vi "WhileLoop.vi"() -> ()   [LabVIEW 2019]
panel:
  in  "milliseconds to wait":u32=500
  out "Waveform Chart":dbl(graph)=0.5543790091498753
  in  "stop":bool
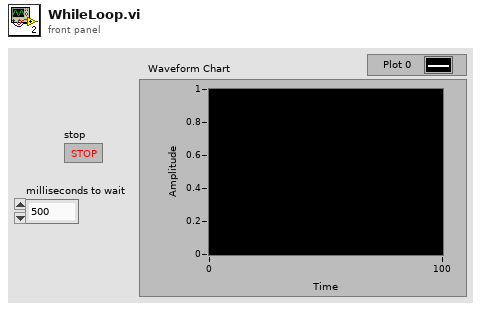
[diagram p1: front panel]
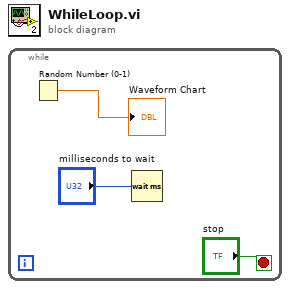
[diagram p0: block diagram]
diagram:
  n1 = while {
    stop <- "stop" stop-if-true
    n2 = Random Number (0-1)() -> (number: 0 to 1=→"Waveform Chart":dbl)
    n3 = Wait (ms)(milliseconds to wait="milliseconds to wait") -> ()  [unwired: 1 out]
  }
